vi "UI Panels - Insert SubPanel.vi"(4 "New Title":string, 6 "Run VI in Panel (T)":bool=TRUE, 7 "Panel index":i32, 8 "error in (no error)":errorcluster, 10 "vi reference":refnum<vi>, 11 "Panels_XControl":refnum<vi>) -> (0 "error out":errorcluster, 3 "Panels_XControl":refnum<vi>)   [LabVIEW 2013, in "UI Panels.lvlib"]
uses:
  UI Panels.lvlib
  Panels_XControl.xctl
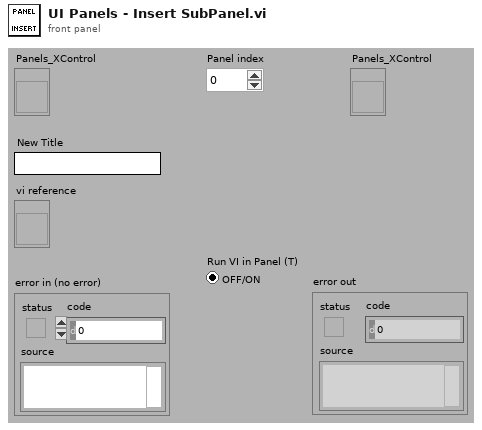
[diagram p1: front panel]
types:
  T1 = enum32{"Bad", "Idle", "Run top level", "Running"}
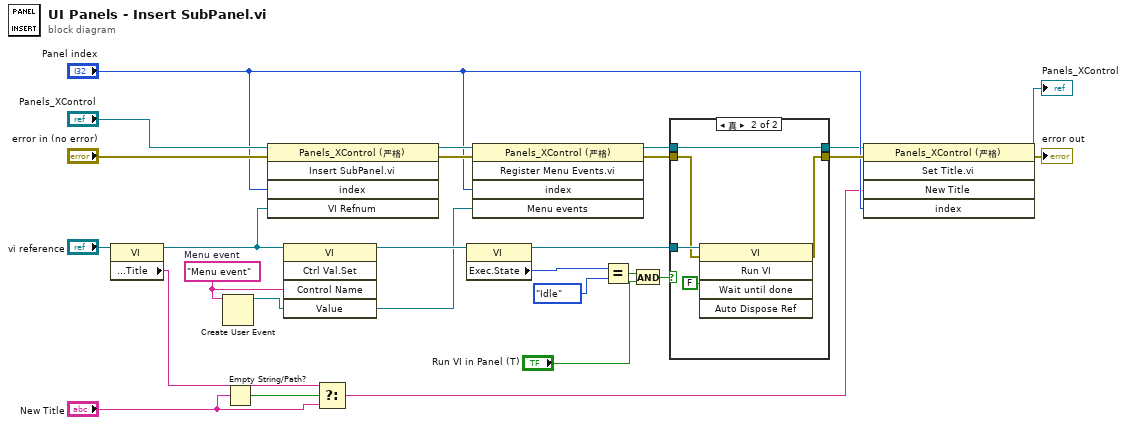
[diagram p0: block diagram]
diagram:
  w20 = "Menu event"  # Menu event
  n1 = property class="VI"(reference="vi reference") -> (reference out=w4:refnum<vi>, "Front Panel.Title"=w10:string)  [unwired: 1 in, 1 out]
  n2 = Create User Event(user event datatype=w20) -> (user event=w17:refnum<user-event>)  [unwired: 1 in, 1 out]
  n3 = Empty String/Path?(string/path="New Title") -> (empty?=w11:bool)
  n4 = invoke on="Invoke Node" class="Panels_XControl (严格)" method="Insert SubPanel.vi"(reference="Panels_XControl", error in="error in (no error)", "index"="Panel index", "VI Refnum"=w4) -> (reference out=w19:refnum<vi>, error out=w18:errorcluster)  [unwired: 1 in, 3 out]
  n5 = invoke class="VI" method="Ctrl Val.Set"(reference=w4, "Control Name"=w20, "Value"=w17) -> (reference out=w21:refnum<vi>)  [unwired: 2 in, 4 out]
  n6 = Select(t=w10, s=w11, f="New Title") -> (s? t:f=w8:string)
  n7 = property class="VI"(reference=w21) -> (reference out=w3:refnum<vi>, "Exec.State"=w2:T1)  [unwired: 1 in, 1 out]
  n8 = invoke class="Panels_XControl (严格)" method="Register Menu Events.vi"(reference=w19, error in=w18, "index"="Panel index", "Menu events"=w17) -> (reference out=w6:refnum<vi>, error out=w16:errorcluster)  [unwired: 1 in, 3 out]
  n9 = Equal?(x=w2, y=T1."Idle" ("Execution:State")) -> (x = y?=w22:bool)
  n10 = And(x=w22, y="Run VI in Panel (T)") -> (x .and. y?=w23:bool)
  n11 = case shown="真" w23 {
    tunnel: w3 -> [_ w32]
    tunnel: w16 -> [w28 w31]
    tunnel: [w28 w30] -> w15
    tunnel: [w27 w29] -> w7
    tunnel: w6 -> [w27 w29]
    frame False {
    }
    frame True {
      n12 = invoke class="VI" method="Run VI"(reference=w32, error in=w31, "Wait until done"=FALSE ("Wait Until Done")) -> (error out=w30:errorcluster)  [unwired: 2 in, 4 out]
    }
  }
  n13 = invoke class="Panels_XControl (严格)" method="Set Title.vi"(reference=w7, error in=w15, "New Title"=w8, "index"="Panel index") -> (reference out=→"Panels_XControl":refnum<vi>, error out=→"error out":errorcluster)  [unwired: 1 in, 3 out]
